vi "Conf Freq and Period.vi"(0 "VISA Resource Name":refnum<visa-resource-name>, 1 "Freq/Period (F:Frequency)":bool, 2 "Set/Check (F:Set)":bool, 3 "Check Parameter(3:Ap Min)":T2(ring)=enum."Frequency-- Aperture Min", 5 "Autorange? (F:Off)":bool, 7 "Voltage Range (6:Maximum)":T1(ring)=enum."Maximum", 9 "Aperture (3:Minimum)":enum16{".01", ".1", "1", "Minimum", "Maximum"}(ring)=enum."Minimum", 11 "error in (no error)":errorcluster, 12 "Channel List(empty)":string, 13 "Low Frequency (1:20 Hz)":u16(ring)=1 items=["3 Hz", "20 Hz", "200 Hz", "MIN", "MAX"]) -> (4 "VISA Resource Name Out":refnum<visa-resource-name>, 8 "Configuration?":string, 15 "error out":errorcluster)   [LabVIEW 2012, in "Agilent 34970.lvlib"]
doc: "This VI configures the instrument for advanced frequency and period measurements.\n\nThis is an advanced measurment configuration VI. For more information on the different ways to take and configure a measurment, refer to the context help and block diagram of \"HP34970A Advanced Scan Example.vi\"."
uses:
  <instrlib>/Agilent 34970/Agilent 34970.lvlib
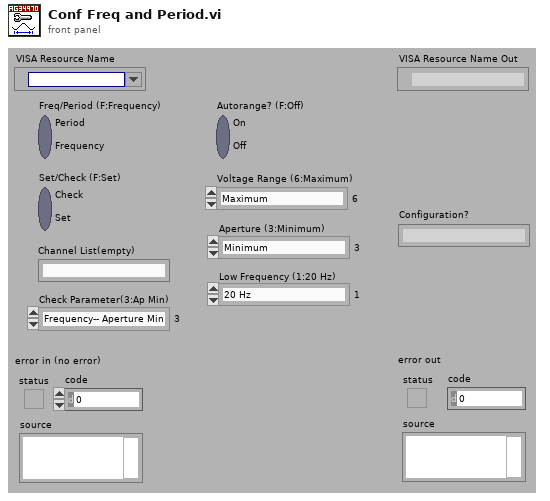
[diagram p1: front panel]
types:
  T1 = enum16{"100 mV", "1 V", "10 V", "100 V", "300 V", "Minimum", "Maximum"}
  T2 = enum16{"Frequency-- Voltage Range", "Frequency-- Voltage Autorange", "Frequency-- Aperture (By Chan)", "Frequency-- Aperture Min", "Frequency-- Aperture Max", "Period-- Voltage Range", "Period-- Voltage Autorange", "Period-- Aperture (By Channel)", "Period-- Aperture Min", "Period-- Aperture Max", "Frequency-- Low Freq (By Channel)", "Frequency-- Low Freq Min", "Frequency-- Low Freq Max"}
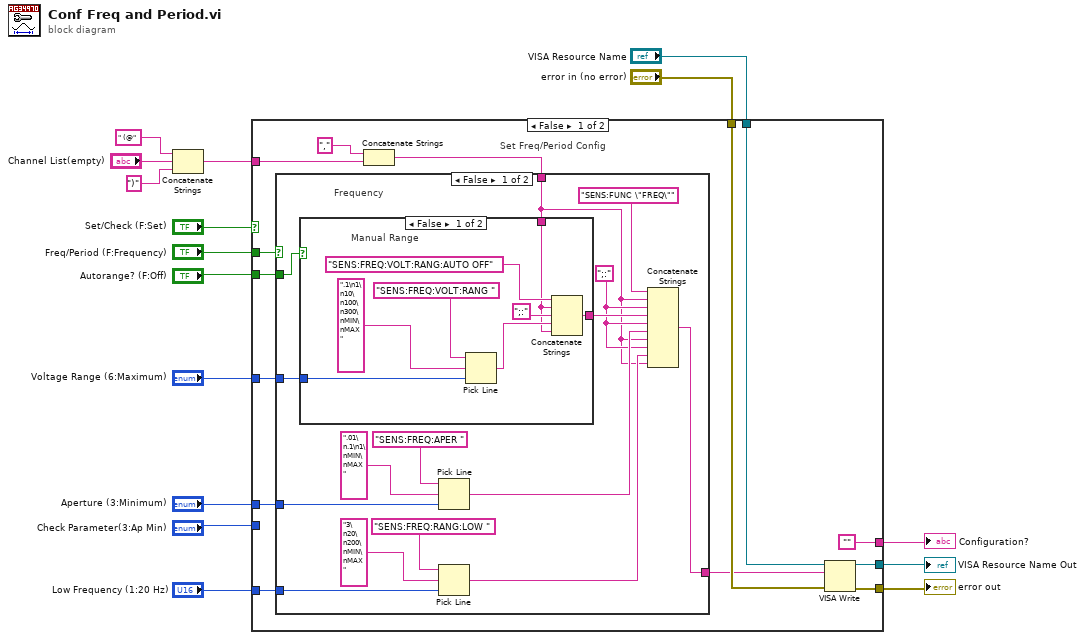
[diagram p0: block diagram]
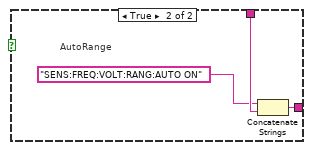
[diagram p2: hidden frame]
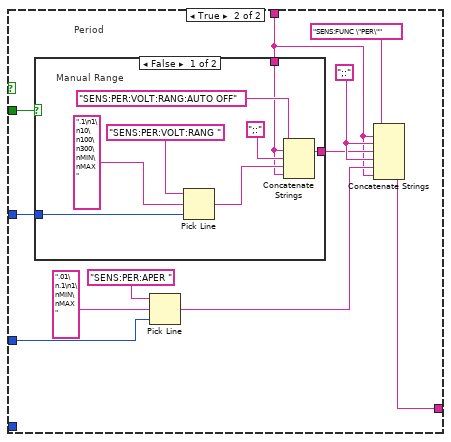
[diagram p3: hidden frame]
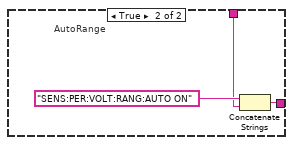
[diagram p4: hidden frame]
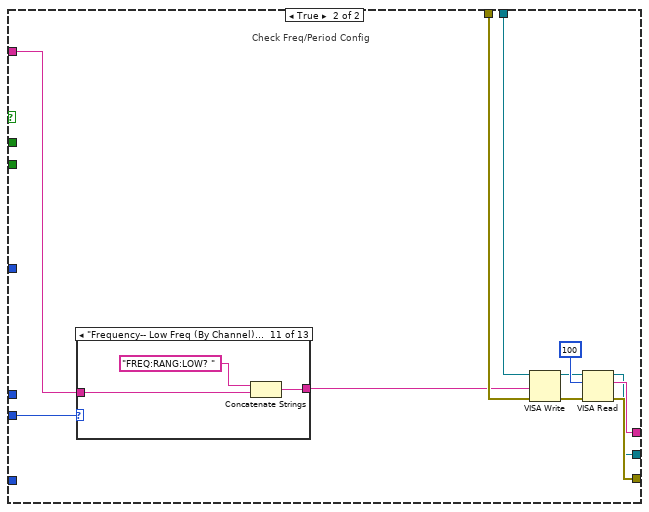
[diagram p5: hidden frame]
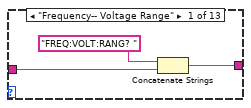
[diagram p6: hidden frame]
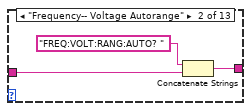
[diagram p7: hidden frame]
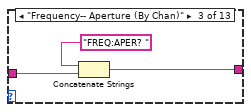
[diagram p8: hidden frame]
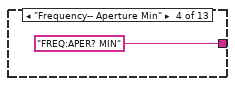
[diagram p9: hidden frame]
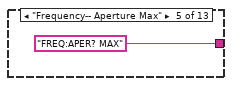
[diagram p10: hidden frame]
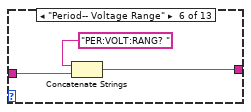
[diagram p11: hidden frame]
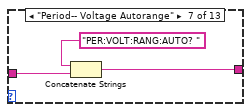
[diagram p12: hidden frame]
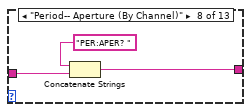
[diagram p13: hidden frame]
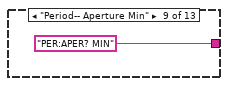
[diagram p14: hidden frame]
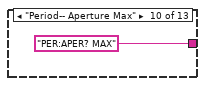
[diagram p15: hidden frame]
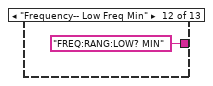
[diagram p16: hidden frame]
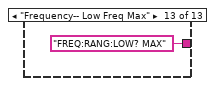
[diagram p17: hidden frame]
diagram:
  n1 = Concatenate Strings(" (@", "Channel List(empty)", ")") -> (w11:string)
  n2 = case shown="False" "Set/Check (F:Set)" {
    tunnel: [w22 w89] -> w5
    tunnel: [w23 w86] -> w4
    tunnel: "Freq/Period (F:Frequency)" -> [w30 _]
    tunnel: w11 -> [w29 w80]
    tunnel: ["" w87] -> w10
    tunnel: "VISA Resource Name" -> [w25 w85]
    tunnel: "error in (no error)" -> [w24 w84]
    tunnel: "Check Parameter(3:Ap Min)" -> [_ w81]
    tunnel: "Autorange? (F:Off)" -> [w21 _]
    tunnel: "Voltage Range (6:Maximum)" -> [w20 _]
    tunnel: "Aperture (3:Minimum)" -> [w19 _]
    tunnel: "Low Frequency (1:20 Hz)" -> [w17 _]
    frame False {
      # "Set Freq/Period Config"
      n3 = Concatenate Strings(",", w29) -> (w27:string)
      n4 = case shown="False" w30 {
        tunnel: w27 -> [w31 w58]
        tunnel: [w45 w57] -> w18
        tunnel: w21 -> [w44 w61]
        tunnel: w20 -> [w43 w60]
        tunnel: w19 -> [w40 w59]
        tunnel: w17 -> [w33 _]
        frame False {
          w36 = ";:"
          # "Frequency"
          n5 = case shown="False" w44 {
            tunnel: w43 -> [w51 _]
            tunnel: w31 -> [w47 w56]
            tunnel: [w46 w54] -> w37
            frame False {
              # "Manual Range"
              n6 = Pick Line(string ("")="SENS:FREQ:VOLT:RANG ", multi-line string=".1\n1\n10\n100\n300\nMIN\nMAX", line index=w51) -> (output string=w48:string)
              n7 = Concatenate Strings("SENS:FREQ:VOLT:RANG:AUTO OFF", w47, ";:", w48, w47) -> (w46:string)
            }
            frame True {
              # "AutoRange"
              n8 = Concatenate Strings("SENS:FREQ:VOLT:RANG:AUTO ON", w56) -> (w54:string)
            }
          }
          n9 = Pick Line(string ("")="SENS:FREQ:APER ", multi-line string=".01\n.1\n1\nMIN\nMAX", line index=w40) -> (output string=w38:string)
          n10 = Pick Line(string ("")="SENS:FREQ:RANG:LOW ", multi-line string="3\n20\n200\nMIN\nMAX", line index=w33) -> (output string=w32:string)
          n11 = Concatenate Strings("SENS:FUNC \"FREQ\"", w31, w36, w37, w36, w38, w31, w36, w32, w31) -> (w45:string)
        }
        frame True {
          w64 = ";:"
          # "Period"
          n12 = case shown="False" w61 {
            tunnel: [w70 w77] -> w62
            tunnel: w60 -> [w69 _]
            tunnel: w58 -> [w68 w76]
            frame False {
              # "Manual Range"
              n13 = Pick Line(string ("")="SENS:PER:VOLT:RANG ", multi-line string=".1\n1\n10\n100\n300\nMIN\nMAX", line index=w69) -> (output string=w71:string)
              n14 = Concatenate Strings("SENS:PER:VOLT:RANG:AUTO OFF", w68, ";:", w71, w68) -> (w70:string)
            }
            frame True {
              # "AutoRange"
              n15 = Concatenate Strings("SENS:PER:VOLT:RANG:AUTO ON", w76) -> (w77:string)
            }
          }
          n16 = Pick Line(string ("")="SENS:PER:APER ", multi-line string=".01\n.1\n1\nMIN\nMAX", line index=w59) -> (output string=w63:string)
          n17 = Concatenate Strings("SENS:FUNC \"PER\"", w58, w64, w62, w64, w63, w58) -> (w57:string)
        }
      }
      n18 = VISA Write(VISA resource name=w25, write buffer=w18, error in (no error)=w24) -> (VISA resource name out=w23:refnum<visa-resource-name>, error out=w22:errorcluster)  [unwired: 1 out]
    }
    frame True {
      # "Check Freq/Period Config"
      n19 = case shown="\"Frequency-- Low Freq (By Channel)\"" w81 {
        tunnel: w80 -> [w92 w94 w97 _ _ w102 w105 w108 _ _ w112 _ _]
        tunnel: [w90 w95 w96 "FREQ:APER? MIN" "FREQ:APER? MAX" w101 w104 w107 "PER:APER? MIN" "PER:APER? MAX" w114 "FREQ:RANG:LOW? MIN" "FREQ:RANG:LOW? MAX"] -> w79
        frame "Frequency-- Voltage Range" {
          n20 = Concatenate Strings("FREQ:VOLT:RANG? ", w92) -> (w90:string)
        }
        frame "Frequency-- Voltage Autorange" {
          n21 = Concatenate Strings("FREQ:VOLT:RANG:AUTO? ", w94) -> (w95:string)
        }
        frame "Frequency-- Aperture (By Chan)" {
          n22 = Concatenate Strings("FREQ:APER? ", w97) -> (w96:string)
        }
        frame "Frequency-- Aperture Min" {
        }
        frame "Frequency-- Aperture Max" {
        }
        frame "Period-- Voltage Range" {
          n23 = Concatenate Strings("PER:VOLT:RANG? ", w102) -> (w101:string)
        }
        frame "Period-- Voltage Autorange" {
          n24 = Concatenate Strings("PER:VOLT:RANG:AUTO? ", w105) -> (w104:string)
        }
        frame "Period-- Aperture (By Channel)" {
          n25 = Concatenate Strings("PER:APER? ", w108) -> (w107:string)
        }
        frame "Period-- Aperture Min" {
        }
        frame "Period-- Aperture Max" {
        }
        frame "Frequency-- Low Freq (By Channel)" {
          n26 = Concatenate Strings("FREQ:RANG:LOW? ", w112) -> (w114:string)
        }
        frame "Frequency-- Low Freq Min" {
        }
        frame "Frequency-- Low Freq Max" {
        }
      }
      n27 = VISA Write(VISA resource name=w85, write buffer=w79, error in (no error)=w84) -> (VISA resource name out=w83:refnum<visa-resource-name>, error out=w82:errorcluster)  [unwired: 1 out]
      n28 = VISA Read(VISA resource name=w83, byte count=u32 100 ("byte count (0)"), error in (no error)=w82) -> (VISA resource name out=w86:refnum<visa-resource-name>, read buffer=w87:string, error out=w89:errorcluster)  [unwired: 1 out]
    }
  }
  "Configuration?" <- w10
  "VISA Resource Name Out" <- w4
  "error out" <- w5
